vi "SchedTestSimple.vi"() -> ()   [LabVIEW 2014]
doc: "This VI is meant for a daily schedule -- turn on/off at certain times."
panel:
  in  "UTC ON hour":i32=22
  in  "UTC OFF hour":i32=8
  in  "stop":bool
  out "ACTIVE":bool
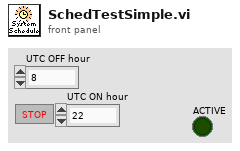
[diagram p1: front panel]
types:
  T1 = typedef "LVDateTimeRec.ctl" = cluster{"fractional second":dbl, "second":i32, "minute":i32, "hour":i32, "day of month":i32, "month":i32, "year":i32, "day of week":i32, "day of year":i32, "DST":i32}
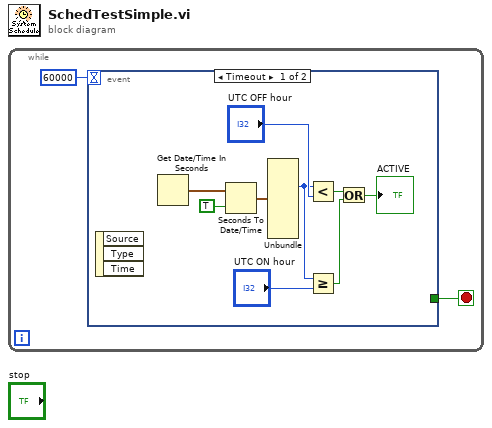
[diagram p0: block diagram]
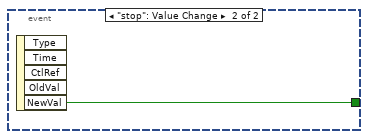
[diagram p2: hidden frame]
diagram:
  n1 = while {
    stop <- w2 stop-if-true
    n2 = event shown="[0] Timeout" {
      selector: _ -> [_ _]
      dyn-events: _ -> [_ _]
      timeout: 60000 -> [_ _]
      tunnel: [_ w12] -> w2
      event Timeout {
        n3 = event-data() -> ()  [unwired: 1 in, 3 out]
        n4 = Get Date/Time In Seconds() -> (seconds since 1Jan1904=w6:timestamp)
        n5 = Seconds To Date/Time(time stamp (now)=w6, to UTC (F)=TRUE) -> (date time rec=w4:T1)
        n6 = Unbundle(w4) -> ("hour"=w3:i32)  [unwired: 9 out]
        n7 = Less?(x=w3, y="UTC OFF hour") -> (x < y?=w10:bool)
        n8 = Greater Or Equal?(x=w3, y="UTC ON hour") -> (x >= y?=w8:bool)
        n9 = Or(x=w10, y=w8) -> (x .or. y?=→"ACTIVE":bool)
      }
      event "stop": Value Change {
        n10 = event-data() -> ("NewVal"=w12:bool)  [unwired: 1 in, 4 out]
      }
    }
  }
